vi "Exemple_Preprocessing_Binarizer.vi"() -> ()   [LabVIEW 2020]
uses:
  Objet/6 - Datasets Transformation/6.3 - Processing Data/Binarizer/Binarizer.lvclass
panel:
  in  "y":string[][](array[string])
  in  "X":string[][](array[string])=[["1", "-1", "2"], ["2", "0", "0"], ["0", "1", "-1"]]
  out "Data":T1
  out "error out":errorcluster
  in  "error in":errorcluster caption="entrée d'erreur"
  in  "Binarizer":cluster{"threshold":dbl, "copy":bool}={"threshold"=0.0, "copy"=TRUE}
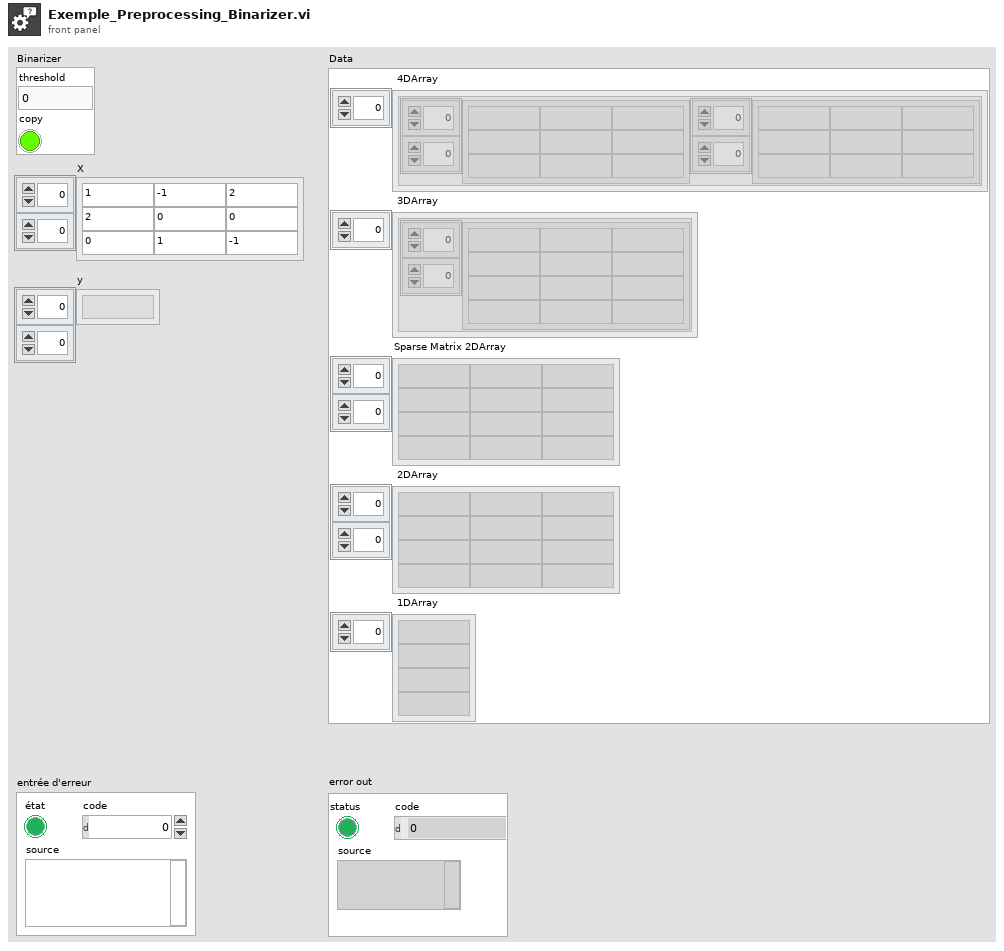
[diagram p1: front panel]
types:
  T1 = cluster{" 4DArray":cluster{"1":string[][], "2":string[][]}[], " 3DArray":cluster{"Tableau":string[][]}[], "Sparse Matrix 2DArray":string[][], " 2DArray":string[][], " 1DArray":string[]}
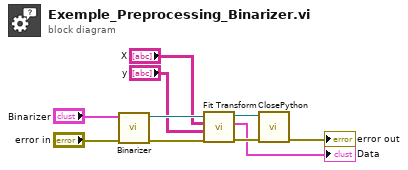
[diagram p0: block diagram]
diagram:
  n1 = call "Binarizer.vi"("error in (no error)"="error in", "Binarizer"="Binarizer") -> ("error out"=w8:errorcluster, "Binarizer en sortie"=w9:refnum<class "Binarizer.lvclass">)  [unwired: 8 in]
  n2 = call-dynamic "Fit Transform.vi"("error in (no error)"=w8, "y"="y", "X"="X", "Binarizer en entrée"=w9) -> ("error out"=w5:errorcluster, "Data"=→"Data":T1, "Binarizer en sortie"=w6:refnum<class "Binarizer.lvclass">)  [unwired: 5 in]
  n3 = call-dynamic "ClosePython.vi"("error in (no error)"=w5, "Scikit-learn en entrée"=w6) -> ("error out"=→"error out":errorcluster)  [unwired: 8 in, 1 out]
